vi "Node PXImc Read.vi"(8 "error in (no error)":errorcluster, 11 "Node Data In":T1) -> (0 "error out":errorcluster, 2 "Readers Data Out":u8[][](array[numeric]), 3 "Node Data In":T1)   [LabVIEW 2016, in "PXImc Router.lvlib"]
uses:
  PXImc Router.lvlib
  Controls/Node Data.ctl
  <vilib>/NI Veristand/VeriStand Data/Byte Buffer/Byte Buffer.lvclass
  Controls/Node/Node - PXImc Parameters.ctl
  Controls/Node/Transfer Data.ctl
  Controls/Node/Node Ch Properties.ctl
  Controls/Data Type.ctl
  <vilib>/pximc/Acquire Read Region (U8).vi
  <resource>/objmgr/pximc.rc
  <vilib>/pximc/nipximc.lvlib
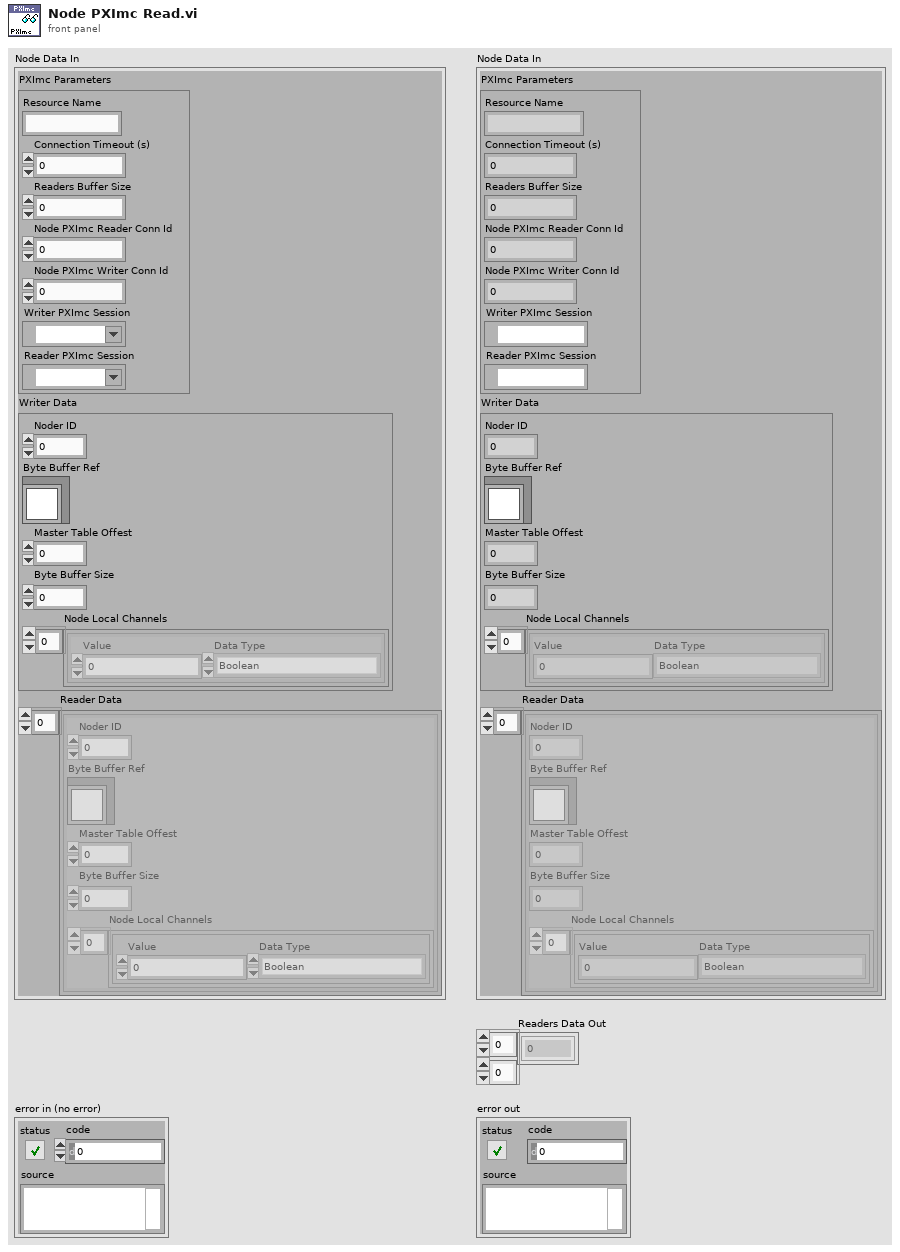
[diagram p1: front panel]
types:
  T1 = typedef "PXImc Router.lvlib/Node Data.ctl" = cluster{"PXImc Parameters":T2, "Writer Data":T3, "Reader Data":T3[]}
  T2 = typedef "PXImc Router.lvlib/Node - PXImc Parameters.ctl" = cluster{"Resource Name":string, "Connection Timeout (s)":dbl, "Readers Buffer Size":u64, "Node PXImc Reader Conn Id":u16, "Node PXImc Writer Conn Id":u16, "Writer PXImc Session":refnum<k21>, "Reader PXImc Session":refnum<k21>}
  T3 = typedef "PXImc Router.lvlib/Transfer Data.ctl" = cluster{"Noder ID":u32, "Byte Buffer Ref":refnum<class "Byte Buffer.lvclass">, "Master Table Offest":u32, "Byte Buffer Size":u32, "Node Local Channels":T4[]}
  T4 = typedef "PXImc Router.lvlib/Node Ch Properties.ctl" = cluster{"Value":dbl, "Data Type":T5}
  T5 = typedef "PXImc Router.lvlib/Data Type.ctl" = enum16{"Boolean", "SGL", "DBL", "I8", "I16", "I32", "I64", "U8", "U16", "U32", "U64"}
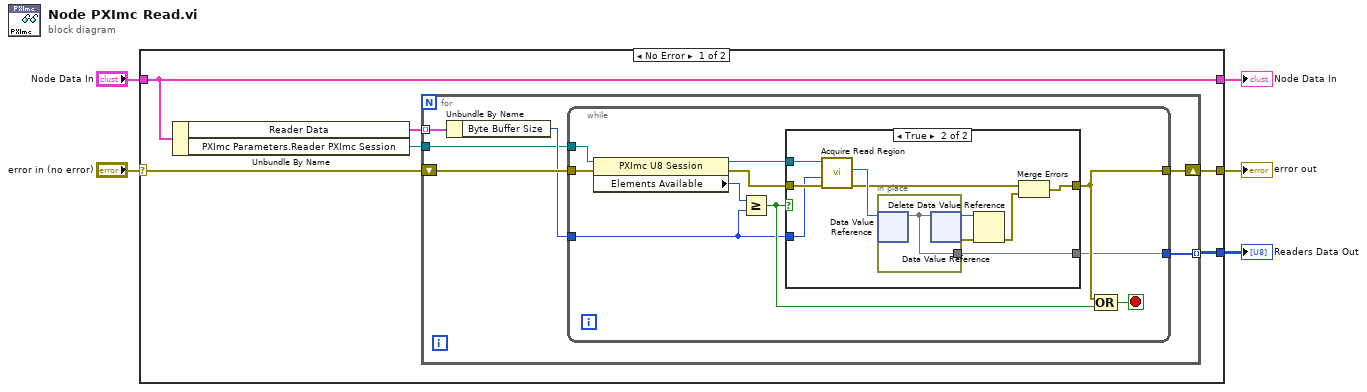
[diagram p0: block diagram]
diagram:
  n1 = case shown="No Error" "error in (no error)" {
    selector: "error in (no error)" -> [w11 w41]
    tunnel: [w10 w41] -> w1
    tunnel: "Node Data In" -> [w7 w40]
    tunnel: [w7 w40] -> w4
    tunnel: [w6 _] -> w5
    frame No Error {
      n2 = Unbundle By Name(w7) -> ("Reader Data"=w9:T3[], "PXImc Parameters.Reader PXImc Session"=w8:refnum<k21>)
      n3 = for {
        shift-right: [w16] -> w10
        shift-left: w11 -> [w17]
        tunnel: w9 -> [w15] mode=indexing
        tunnel: w8 -> [w13]
        tunnel: [w12] -> w6 mode=indexing
        n4 = Unbundle By Name(w15) -> ("Byte Buffer Size"=w14:u32)
        n5 = while {
          tunnel: w17 -> [w25]
          tunnel: [w21] -> w16
          tunnel: [w20] -> w12
          tunnel: w14 -> [w18]
          tunnel: w13 -> [w19]
          stop <- w22 stop-if-true
          n6 = property class="PXImc U8 Session"(reference=w19, error in=w25) -> (reference out=w26:refnum<k21>, error out=w24:errorcluster, "Elements Available"=w27:u64)
          n7 = Greater Or Equal?(x=w27, y=w18) -> (x >= y?=w23:bool)
          n8 = case shown="True" w23 {
            tunnel: w24 -> [w28 w37]
            tunnel: [w28 w31] -> w21
            tunnel: w26 -> [_ w36]
            tunnel: w18 -> [_ w30]
            tunnel: [_ w29] -> w20
            frame False {
            }
            frame True {
              n9 = call-poly <vilib>:"Acquire Read Region.vi"("error in (no error)"=w37, "number of elements"=w30, "session in"=w36) -> ("error out"=w32:errorcluster, "read region reference"=w38:refnum<data-value>)  [unwired: 5 in, 2 out]
              n10 = in-place {
                in-place-border: [w39] -> w29
                n11 = in-place-dvr #1(w38) -> (w39:u8[])  [unwired: 1 out]
                n12 = in-place-dvr #1(w39) -> (w35:refnum<data-value>, w34:errorcluster)
              }
              n13 = Delete Data Value Reference(data value reference=w35, error in=w34) -> (error out=w33:errorcluster)  [unwired: 1 out]
              n14 = Merge Errors(w32, w33) -> (w31:errorcluster)
            }
          }
          n15 = Compound Arithmetic op=OR(w21, w23) -> (w22:bool)
        }
      }
    }
    frame Error {
    }
  }
  "Readers Data Out" <- w5
  "Node Data In" <- w4
  "error out" <- w1
